vi "Stop Command.vi"(8 "error in (no error)":errorcluster, 11 "Command Actor in":refnum<class "Command Actor.lvclass">) -> (0 "error out":errorcluster, 3 "Command Actor out":refnum<class "Command Actor.lvclass">)   [LabVIEW 2014, in "Robot Actor Framework.lvlib" / "Command Actor.lvlib" / "Command Actor.lvclass"]
uses:
  Command Actor.lvclass
  Command States.ctl
  Command Actor.lvclass/Command Actor.ctl
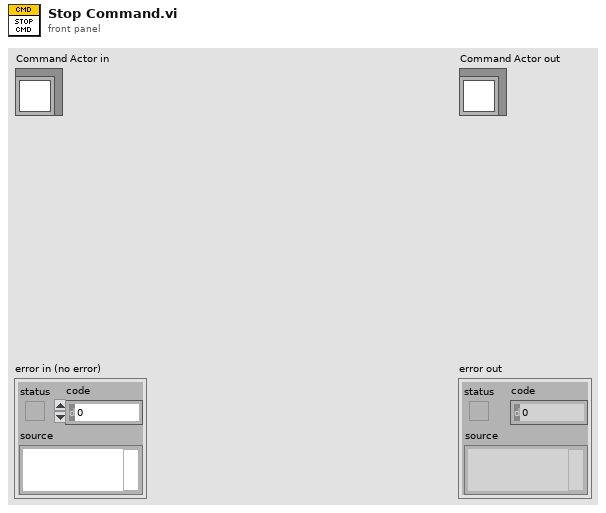
[diagram p1: front panel]
types:
  T1 = typedef "Robot Actor Framework.lvlib/Command Actor.lvlib/Command Actor.lvclass/Command States.ctl" = enum16{"Unknown", "Started", "Stopped", "Finished"}
  T2 = enum16{"Critical", "Error", "Warning", "Informational", "Debug"}
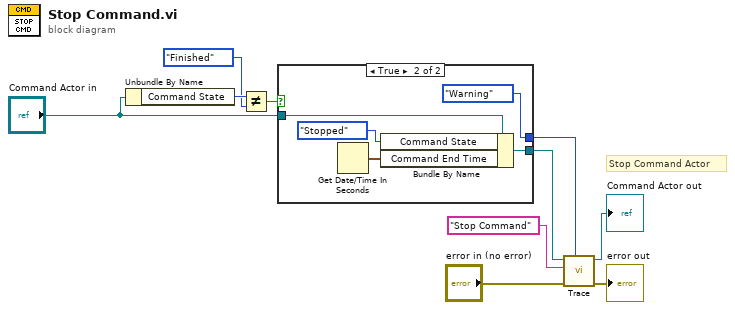
[diagram p0: block diagram]
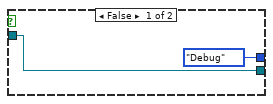
[diagram p2: hidden frame]
diagram:
  # "Stop Command Actor"
  n1 = Unbundle By Name("Command Actor in") -> ("Command State"=w4:T1)
  n2 = Not Equal?(x=w4, y=Command_States."Finished") -> (x != y?=w2:bool)
  n3 = case shown="True" w2 {
    tunnel: [w12 w15] -> w9
    tunnel: "Command Actor in" -> [w12 w14]
    tunnel: [T2."Debug" ("Trace Level") T2."Warning" ("Trace Level")] -> w1
    frame False {
    }
    frame True {
      n4 = Get Date/Time In Seconds() -> (seconds since 1Jan1904=w16:timestamp)
      n5 = Bundle By Name(cluster=w14, "Command State"=Command_States."Stopped", "Command End Time"=w16) -> (w15:refnum<class "Command Actor.lvclass">)
    }
  }
  n6 = call-dynamic "Trace.vi"("Trace Level"=w1, "error in (no error)"="error in (no error)", "Command Action"="Stop Command", "Command Actor in"=w9) -> ("error out"=→"error out":errorcluster, "Command Actor out"=→"Command Actor out":refnum<class "Command Actor.lvclass">)  [unwired: 6 in]
